vi "Remove error (SubVI).vi"(11 "X axis in":dbl) -> (3 "X axis out":dbl)   [LabVIEW 2014]
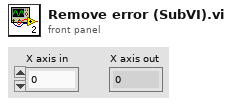
[diagram p1: front panel]
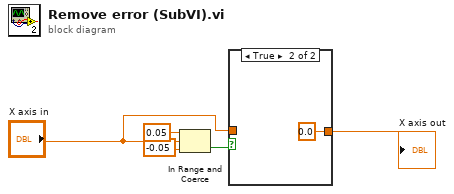
[diagram p0: block diagram]
diagram:
  n1 = In Range and Coerce(upper limit=0.05, x="X axis in", lower limit=-0.05) -> (In Range?=w1:bool)  [unwired: 1 out]
  n2 = case shown="True" w1 {
    tunnel: "X axis in" -> [w6 _]
    tunnel: [w6 0.0 ("X axis")] -> w5
    frame False {
    }
    frame True {
    }
  }
  "X axis out" <- w5
